vi "Write Reply State.vi"(8 "error in (no error)":errorcluster, 10 "Reply State":T1, 11 "Scenarios Class in":refnum<class "Scenarios Class.lvclass">) -> (0 "error out":errorcluster, 3 "Scenarios Class out":refnum<class "Scenarios Class.lvclass">)   [LabVIEW 2020, in "SECS Scenarios.lvlib" / "Scenarios Class.lvclass"]
uses:
  Scenarios Class.lvclass
  Reply State.ctl
  Scenarios Class.lvclass/Scenarios Class.ctl
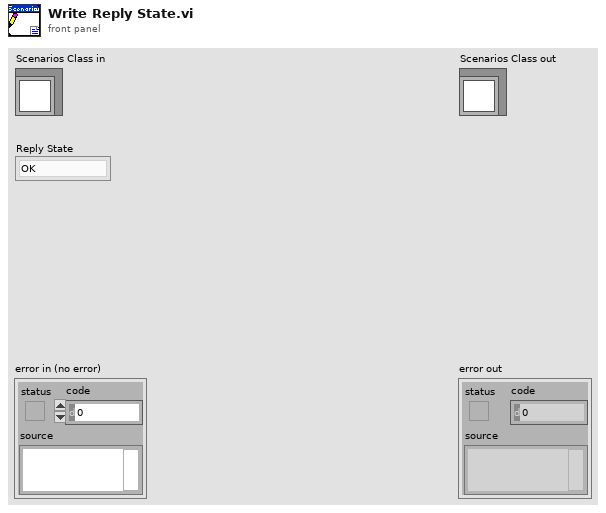
[diagram p1: front panel]
types:
  T1 = typedef "SECS Scenarios.lvlib/Scenarios Class.lvclass/Reply State.ctl" = enum16{"OK", "Illegal Data", "Unknown Stream", "Unknown Function", "Off-Line", "T3 Timeout", "Inner-Timeout"}
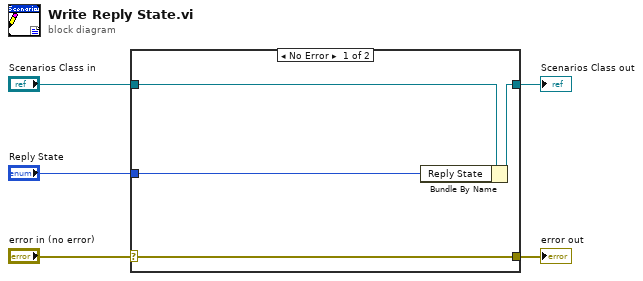
[diagram p0: block diagram]
diagram:
  n1 = case shown="No Error" "error in (no error)" {
    selector: "error in (no error)" -> [w9 w10]
    tunnel: [w9 w10] -> w4
    tunnel: [w7 w11] -> w2
    tunnel: "Scenarios Class in" -> [w8 w11]
    tunnel: "Reply State" -> [w6 _]
    frame No Error {
      n2 = Bundle By Name(cluster=w8, "Reply State"=w6) -> (w7:refnum<class "Scenarios Class.lvclass">)
    }
    frame Error {
    }
  }
  "error out" <- w4
  "Scenarios Class out" <- w2
